vi "cluster_v18.vi"() -> ()   [LabVIEW 2009]
panel:
  out "Mixed Signal Graph":cluster{dbl[], i32[], dbl[]}(graph)={[0.0, 0.3499745141815259, 0.6556837070328476, 0.8784610039697877, 0.9901291856966776, 0.9765642867640316, 0.8394820167042125, 0.5962207544190748, 0.2775485630272303, -0.07622840265330541, -0.42036388130776986, -0.7113310819085673, -0.9123280199990134, -0.9979322899740363, -0.9573165305140726, -0.7956178860988287, -0.5332882529769173, -0.20350749149254924, 0.15201321429916073, 0.48830705211985215, 0.762839053881022, 0.940885984658543, 0.9999281914966702, 0.9324979241683725, 0.7471238678484814, 0.4672524217368729, 0.12828216199059414, -0.22691342529054118, -0.553408649323472, -0.8099078859442701, -0.9639687124338816, -0.9961052756440918, -0.9022528930357296, -0.6942821600533817, -0.3984975387355785, -0.0523103284101769, 0.3004931736797289, 0.6152898314096268, 0.8522636734917913, 0.9814418795019901, 0.9864857888629719, 0.866757440067321, 0.6374002610419791, 0.3274237048115151, -0.02396591127704347, -0.37232428160151987, -0.673590497222469, -0.8896599382318261, -0.9932038053932101, -0.9711257092098341, -0.8262181216541254, -0.5768091799658464, -0.2544445153241085, 0.1001026876886631, 0.4419887469409566, 0.7279713814726488, 0.9218790625025379, 0.9991860446938376, 0.9501144206015728, 0.7808708456266942, 0.5128615105795664, 0.17998465334502745, -0.17565694301188872, -0.5090811757859506, -0.7781160290018373, -0.9487335556403842, -0.9993537853460852, -0.9235741926694184, -0.7309794984519833, -0.44592937941471184, -0.10447741832750393, 0.25018900926116905, 0.5732111415098479, 0.8237326363097475, 0.9700671450323871, 0.9937060512276371, 0.8916594692431826, 0.6768344096159361, 0.3764022802880389, 0.028362204634856763, -0.32326516680965195, -0.634005456755791, -0.8645557496273418, -0.9857556855032394, -0.982275707831935, -0.8545559696062897, -0.6187506621278885, -0.3046848077453163, 0.04791805539864621, 0.3944601683056979, 0.6911103451017604, 0.9003478096547577, 0.9957078817452769, 0.965129271016138, 0.8124796077515652, 0.5570662589784359, 0.23119430263051355, -0.12391946899526739, -0.4633597132872808, -0.7441934997687913, -0.9309005339747628, -0.9998658195873557, -0.9423665199297022, -0.7656752359269327, -0.49214015622049784, -0.15635842348120804, 0.19919976605026873, 0.5295628590938253, 0.792946017392278, 0.9560361290971414, 0.9982053030110349, 0.9141199163760451, 0.7144152197825688, 0.4243501741196086, 0.08061265788301211, -0.2733208728057181, -0.5926843540458776, -0.8370841956033501, -0.9756083250808334, -0.9907359949529021], [0, 0, 0, 0, 0, 0, 0, 0, 0, 0, 0, 0, 0, 0, 0, 0, 0, 0, 0, 0, 0, 0, 0, 0, 0, 0, 0, 0, 0, 0, 0, 0, 0, 0, 0, 0, 0, 0, 0, 0, 0, 0, 0, 0, 0, 0, 0, 0, 0, 0, 0, 0, 0, 0, 0, 0, 0, 0, 0, 0, 0, 0, 0, 0, 0, 0, 0, 0, 0, 0, 0, 0, 0, 0, 0, 0, 0, 0, 0, 0, 0, 0, 0, 0, 0, 0, 0, 0, 0, 0, 0, 0, 0, 0, 0, 0, 0, 0, 0, 0, 0, 0, 0, 0, 0, 0, 0, 0, 0, 0, 0, 0, 0, 0, 0, 0, 0, 0, 0, 0], [1.0, 0.9975385883404528, 0.9901664704565271, 0.9779199379820526, 0.9608592784326729, 0.9390684784210568, 0.9126548102056431, 0.8817483036082656, 0.8465011059003136, 0.8070867328085964, 0.7636992143280776, 0.7165521395464904, 0.665877605182997, 0.6119250730170461, 0.5549601418321084, 0.49526323991979193, 0.43312824458090793, 0.36886103541944265, 0.30277798855130955, 0.2352044191406274, 0.16647297993064597, 0.09692202365306263, 0.02689393737730619, -0.043266543000513295, -0.11321402983151348, -0.18260418399641046, -0.25109541002616553, -0.3183505377161264, -0.38403848195537227, -0.4478358726002184, -0.5094286463683013, -0.5685135929166281, -0.6247998474925224, -0.6780103228094141, -0.7278830730985933, -0.7741725836219485, -0.8166509792976461, -0.8551091464888964, -0.8893577624334401, -0.9192282272460591, -0.9445734939060215, -0.9652687921435852, -0.9812122426619904, -0.9923253586712384, -0.9985534322646911, -0.9998658037364295, -0.9962560125135694, -0.9877418289605197, -0.9743651668986184, -0.9561918772717953, -0.9333114239740101, -0.9058364434343088, -0.8739021901275836, -0.8376658707406907, -0.7973058702717063, -0.7530208738720977, -0.7050288887548264, -0.6535661709833582, -0.5988860624248019, -0.5412577435926603, -0.4809649085187205, -0.41830436817745786, -0.35358458933805303, -0.28712417603698254, -0.21925030114664143, -0.15029709576109723, -0.08060400432774815, -0.010514113622282068, 0.05962753620690428, 0.12947565021039026, 0.19868637846376563, 0.2669190087800532, 0.33383764397560883, 0.3991128554326099, 0.46242330481793775, 0.5234573259750145, 0.5819144592012306, 0.6375069303579729, 0.6899610675318648, 0.7390186482732437, 0.7844381707796576, 0.8259960427665703, 0.8634876821726716, 0.8967285242812227, 0.9255549302995452, 0.9498249929238866, 0.9694192349240036, 0.9842411973084585, 0.9942179141751899, 0.9993002719097585, 0.9994632509629925, 0.9947060490178082, 0.985052084938875, 0.970548883485682, 0.9512678413565451, 0.9273038757152737, 0.8987749569307448, 0.8658215278296193, 0.8286058123211203, 0.78731101679739, 0.7421404282407891, 0.6933164134780023, 0.6410793245074354, 0.5856863152887941, 0.5274100758195747, 0.46653748973038545, 0.403368222007519, 0.33821324379517315, 0.2713933015394459, 0.20323733801025431, 0.13408087297419521, 0.06426435149001425, -0.005868532042269118, -0.07597252582816506, -0.14570252029230366, -0.2147152469918956, -0.28267096846663253, -0.3492351507061709, -0.41408011000196393, -0.47688662607626775]}
  in  "Nr de perioade cosinus":dbl(knob)=1.3402864406190487 scale=0.0..25.0
  in  "stop":bool
  in  "Nr de perioade sinus":dbl(knob)=6.8285854321978485 scale=0.0..25.0
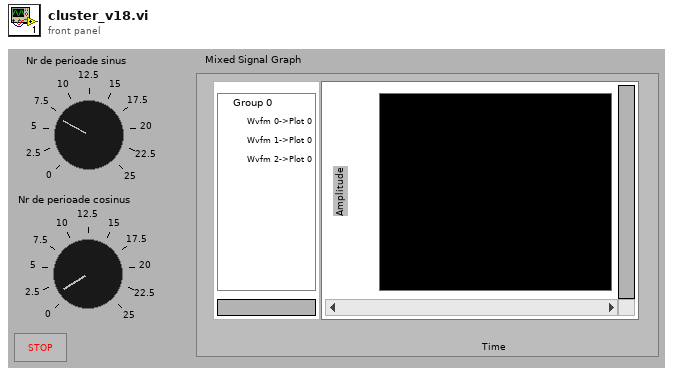
[diagram p1: front panel]
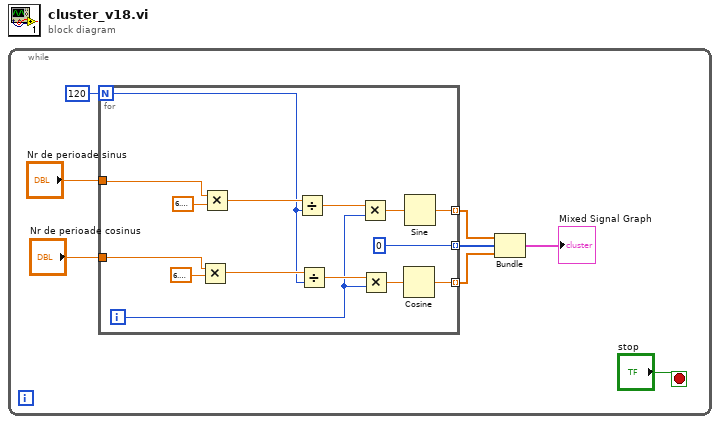
[diagram p0: block diagram]
diagram:
  n1 = while {
    stop <- "stop" stop-if-true
    n2 = for {
      N: 120 -> [w15]
      tunnel: [w23] -> w4 mode=indexing
      tunnel: "Nr de perioade sinus" -> [w20]
      tunnel: "Nr de perioade cosinus" -> [w17]
      tunnel: [w11] -> w2 mode=indexing
      tunnel: [0] -> w3 mode=indexing
      i -> [w13]
      n3 = Multiply(x=w17, y=6.283185307179586) -> (x*y=w16:dbl)
      n4 = Multiply(x=w20, y=6.283185307179586) -> (x*y=w21:dbl)
      n5 = Divide(x=w21, y=w15) -> (x/y=w22:dbl)
      n6 = Divide(x=w16, y=w15) -> (x/y=w14:dbl)
      n7 = Multiply(x=w22, y=w13) -> (x*y=w10:dbl)
      n8 = Multiply(x=w14, y=w13) -> (x*y=w12:dbl)
      n9 = Cosine(x=w12) -> (cos(x)=w11:dbl)
      n10 = Sine(x=w10) -> (sin(x)=w23:dbl)
    }
    n11 = Bundle(w4, w3, w2) -> (→"Mixed Signal Graph":cluster{dbl[], i32[], dbl[]})  [unwired: 1 in]
  }
